vi "Test shm issue Command fault LV.vi"(8 "error in (no error)":errorcluster, 11 "command_fault_Ctl":cluster{"ignored":u8}) -> (0 "error out":errorcluster, 2 "function return":i32, 3 "command_fault_Ctl out":cluster{"ignored":u8})   [LabVIEW 2018, in "SALLV_Test.lvlib"]
doc: "int Test_shm_issueCommand_faultLV(Test_command_faultLV *command_fault_Ctl );"
uses:
  SALLV_Test.lvlib
  SALLV_Test.so
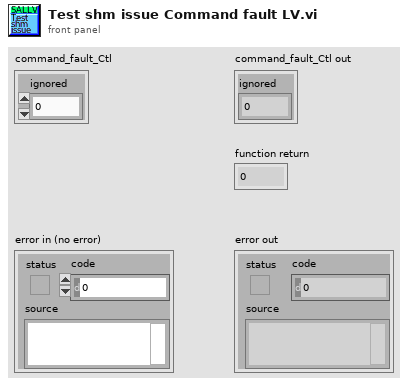
[diagram p1: front panel]
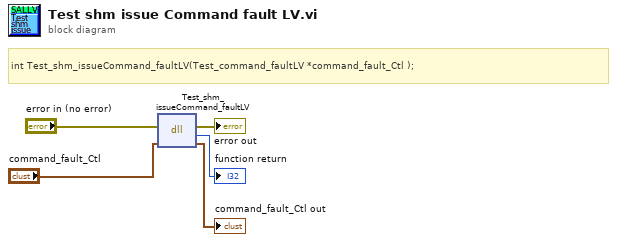
[diagram p0: block diagram]
diagram:
  # "int Test_shm_issueCommand_faultLV(Test_command_faultLV *command_fault_Ctl );"
  n1 = dll-call lib="home/ttsai/Documents/salLabVIEWtestData/SALLV_Test.*" fn="Test_shm_issueCommand_faultLV"(error in="error in (no error)", "command_fault_Ctl"="command_fault_Ctl") -> (error out=→"error out":errorcluster, →"function return":i32, "command_fault_Ctl"=→"command_fault_Ctl out":cluster{"ignored":u8})  [unwired: 2 in, 1 out]
